vi "Read_Endpoint_State.vi"(0 "error in":errorcluster, 2 "Side":T3, 3 "node":string) -> (1 "error out":errorcluster, 4 "Endpoint State":T2)   [LabVIEW 2010]
uses:
  ROS/Code/SubVIs/_ROSDirection.ctl
  ROS/Code/Console/Servers/ServerSubs/TopicDef.ctl
  ROS/Code/SubVIs/BaxterSide.ctl
panel:
  out "Orientation":T1
  out "Reply":string
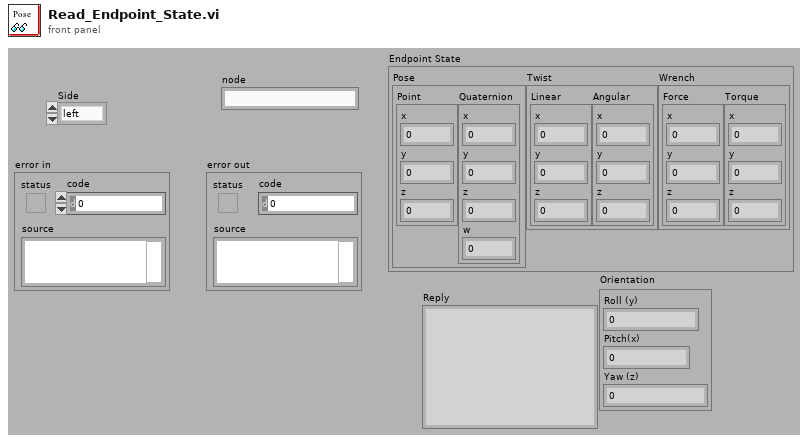
[diagram p1: front panel]
types:
  T1 = cluster{"Roll (y)":dbl, "Pitch(x)":dbl, "Yaw (z)":dbl}
  T2 = cluster{"Pose":cluster{"Point":cluster{"x":dbl, "y":dbl, "z":dbl}, "Quaternion":cluster{"x":dbl, "y":dbl, "z":dbl, "w":dbl}}, "Twist":cluster{"Linear":cluster{"x":dbl, "y":dbl, "z":dbl}, "Angular":cluster{"x":dbl, "y":dbl, "z":dbl}}, "Wrench":cluster{"Force":cluster{"x":dbl, "y":dbl, "z":dbl}, "Torque":cluster{"x":dbl, "y":dbl, "z":dbl}}}
  T3 = typedef "BaxterSide.ctl" = enum16{"left", "right"}
  T4 = typedef "TopicDef.ctl" = cluster{"Topic":string, "Type":string, "Action":T5, "Update (ms)":u16, "write queue":u16}
  T5 = typedef "_ROSDirection.ctl" = enum16{"Node", "Publisher", "Subscriber", "Service Client"}
  T6 = typedef "_ROSControl.ctl" = cluster{"topic port":u16, "Node":string, "topic":string, "type":string, "node port":u32, "error ":errorcluster, "Direction":T5, "APIs":string[], "Update (ms)":u16, "write queue":u16}
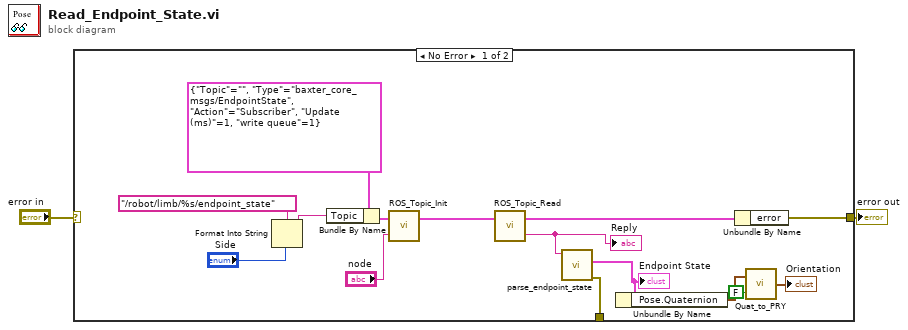
[diagram p0: block diagram]
diagram:
  n1 = case shown="No Error" "error in" {
    selector: "error in" -> [_ w18]
    tunnel: [w17 w18] -> w2
    tunnel: [w12 _] -> _
    frame No Error {
      n2 = Format Into String(format string="/robot/limb/%s/endpoint_state" ("topic"), "Side") -> (resulting string=w5:string)  [unwired: 2 in, 1 out]
      n3 = Bundle By Name(cluster=T4 {"Topic"="", "Type"="baxter_core_msgs/EndpointState", "Action"=enum."Subscriber", "Update (ms)"=1, "write queue"=1} ("Definitions"), "Topic"=w5) -> (w3:T4)
      n4 = call "ROS_Topic_Init.vi"("node"="node", "Definitions"=w3) -> ("ROS out"=w15:T6)  [unwired: 1 in]
      n5 = call "ROS_Topic_Read.vi"("ROS in"=w15) -> ("Reply"=w13:string, "ROS out"=w14:T6)  [unwired: 1 in]
      "Reply" <- w13
      n6 = call "parse_endpoint_state.vi"("msg in"=w13) -> ("error out"=w12:errorcluster, "Endpoint State"=w11:T2)  [unwired: 4 in, 1 out]
      "Endpoint State" <- w11
      n7 = Unbundle By Name(w11) -> ("Pose.Quaternion"=w10:cluster{"x":dbl, "y":dbl, "z":dbl, "w":dbl})
      n8 = Unbundle By Name(w14) -> ("error"=w17:errorcluster)
      n9 = call "Quat_to_PRY.vi"("toDegrees? (T)"=FALSE, "Quaternion"=w10) -> ("Orientation"=→"Orientation":T1)
    }
    frame Error {
    }
  }
  "error out" <- w2
